vi "destroyNetworkConnection.vi"(8 "error in (no error)":errorcluster, 11 "BuildWorker in":refnum<class "BuildWorker.lvclass">) -> (0 "error out":errorcluster, 3 "BuildWorker out":refnum<class "BuildWorker.lvclass">)   [LabVIEW 2017, in "BuildWorker.lvlib" / "BuildWorker.lvclass"]
uses:
  BuildWorker.lvclass
  BuildWorker.lvclass/BuildWorker.ctl
  <vilib>/ActorFramework/Message Enqueuer/Message Enqueuer.lvclass/Message Enqueuer.ctl
  <vilib>/ActorFramework/Message Enqueuer/Enqueue.vi
  <vilib>/ActorFramework/Stop Msg/Stop Msg.lvclass
  C:/Program Files (x86)/National Instruments/LabVIEW 2017/vi.lib/ActorFramework/Message/Message.lvclass
  <vilib>/ActorFramework/Message Priority Queue/Priority Enqueue.vi
  BuildWorker Messages/Send Worker Status Update Msg/Send Worker Status Update Msg.lvclass
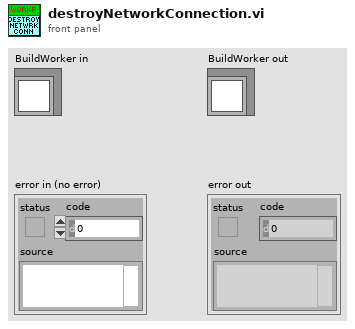
[diagram p1: front panel]
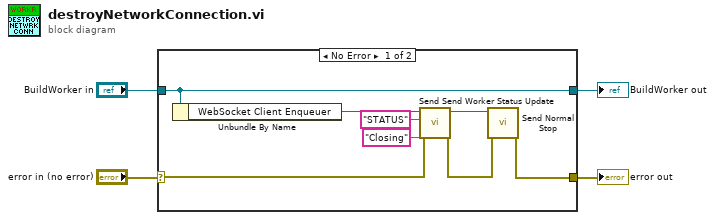
[diagram p0: block diagram]
diagram:
  n1 = case shown="No Error" "error in (no error)" {
    selector: "error in (no error)" -> [w6 w14]
    tunnel: [w11 w14] -> w3
    tunnel: [w12 w13] -> w1
    tunnel: "BuildWorker in" -> [w12 w13]
    frame No Error {
      n2 = Unbundle By Name(w12) -> ("WebSocket Client Enqueuer"=w8:refnum<class "Message Enqueuer.lvclass">)
      n3 = call "Send Send Worker Status Update.vi"("error in (no error)"=w6, "Status"="Closing", "Operation"="STATUS", "Message Enqueuer in"=w8) -> ("error out"=w5:errorcluster, "Message Enqueuer out"=w7:refnum<class "Message Enqueuer.lvclass">)  [unwired: 6 in]
      n4 = call <vilib>:"Send Normal Stop.vi"("error in (no error)"=w5, "Message Enqueuer"=w7) -> ("error out"=w11:errorcluster)  [unwired: 9 in]
    }
    frame Error {
    }
  }
  "error out" <- w3
  "BuildWorker out" <- w1
